vi "SETUPdll.vi"(8 "error in (no error)":errorcluster, 11 "Inputs":T1={"ncomp - Number of Components"=1, "hfld - Fluid/Mixture Components"="", "hfm - Mixture Coefficients "="", "hrf - Reference state"="DEF"}) -> (0 "error out":errorcluster, 2 "herr out":string, 3 "ierr out":i32=101)   [LabVIEW 2021]
doc: "INITIALIZATION SUBROUTINES\n\nsubroutine SETUP (ncomp,hfiles,hfmix,hrf,ierr,herr)\n\ndefine models and initialize arrays\n\nA call to this routine is required.\n\nINPUTS:\nncomp -- number of components (1 for pure fluid) [integer]\n if called with ncomp=-1, the version number*10000 will be returned in ierr\nhfiles -- array of file names specifying fluid/mixture components\n [character*255 variable] for each of the ncomp components;\n e.g., :fluids:r134a.fld (Mac) or fluids\\r134a.fld (DOS) or\n [full_path]/fluids/r134a.fld (UNIX)\nhfmix -- mixture coefficients [character*255]\n file name containing coefficients for mixture model,\n if applicable\n e.g., fluids\\hmx.bnc\nhrf -- reference state for thermodynamic calculations [character*3]\n 'DEF': default reference state as specified in fluid file\n is applied to each pure component\n 'NBP': h,s = 0 at pure component normal boiling point(s)\n 'ASH': h,s = 0 for sat liquid at -40 C (ASHRAE convention)\n 'IIR': h = 200, s = 1.0 for sat liq at 0 C (IIR convention)\n other choices are possible, but these require a separate\n call to SETREF\nOUTPUTS:\nierr -- error flag: 0 = successful\n 101 = error in opening file\n 102 = error in file or premature end of file\n -103 = unknown model encountered in file\n 104 = error in setup of model\n 105 = specified model not found\n 111 = error in opening mixture file\n 112 = mixture file of wrong type\n 114 = nc<>nc from setmod\n -117 = binary pair not found, all parameters will be estimated\n 117 = No mixture data are available, mixture is outside the\n range of the model and calculations will not be made\nherr -- error string (character*255 variable if ierr<>0)\n [fluid parameters, etc. returned via various common blocks]\nhfld_length -- length of variable hfld (default: 10000)\nhfm_length -- length of variable hfm (default: 255)\nhrf_length -- length of variable hrf (default: 3)\nherr_length -- : length of variable herr (default: 255)"
uses:
  REFPROP.dll
panel:
  # "REFPROP-SETUP_dll.vi"
  # "void  SETUPdll(int32_t *ncomp, CStr hfiles, CStr hfmix, CStr hrf, int32_t *ierr, CStr herr, int32_t hfile_Lengh, int32_t hfmix_length, int32_t hrf_length, int32_t herr_length)"
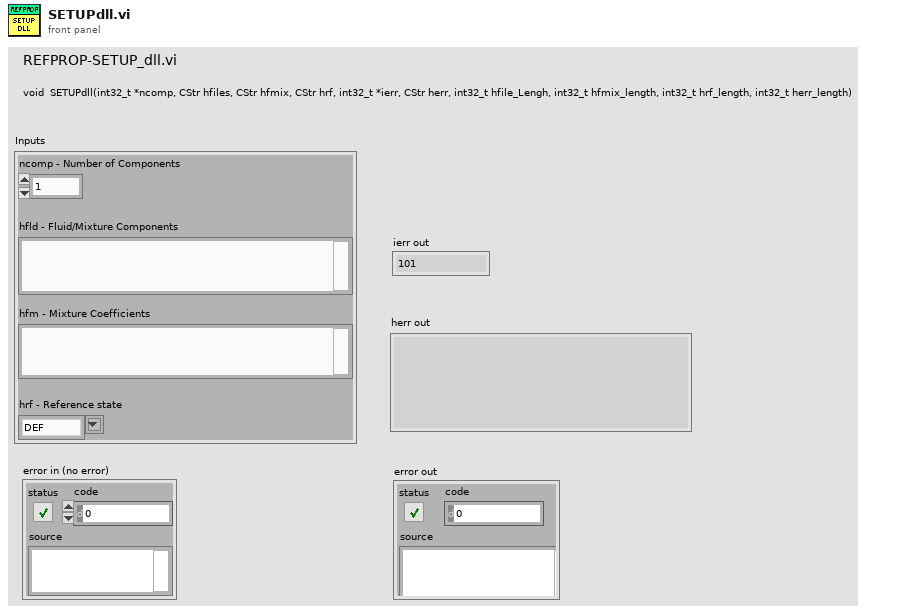
[diagram p1: front panel]
types:
  T1 = cluster{"ncomp - Number of Components":i32, "hfld - Fluid/Mixture Components":string, "hfm - Mixture Coefficients ":string, "hrf - Reference state":string}
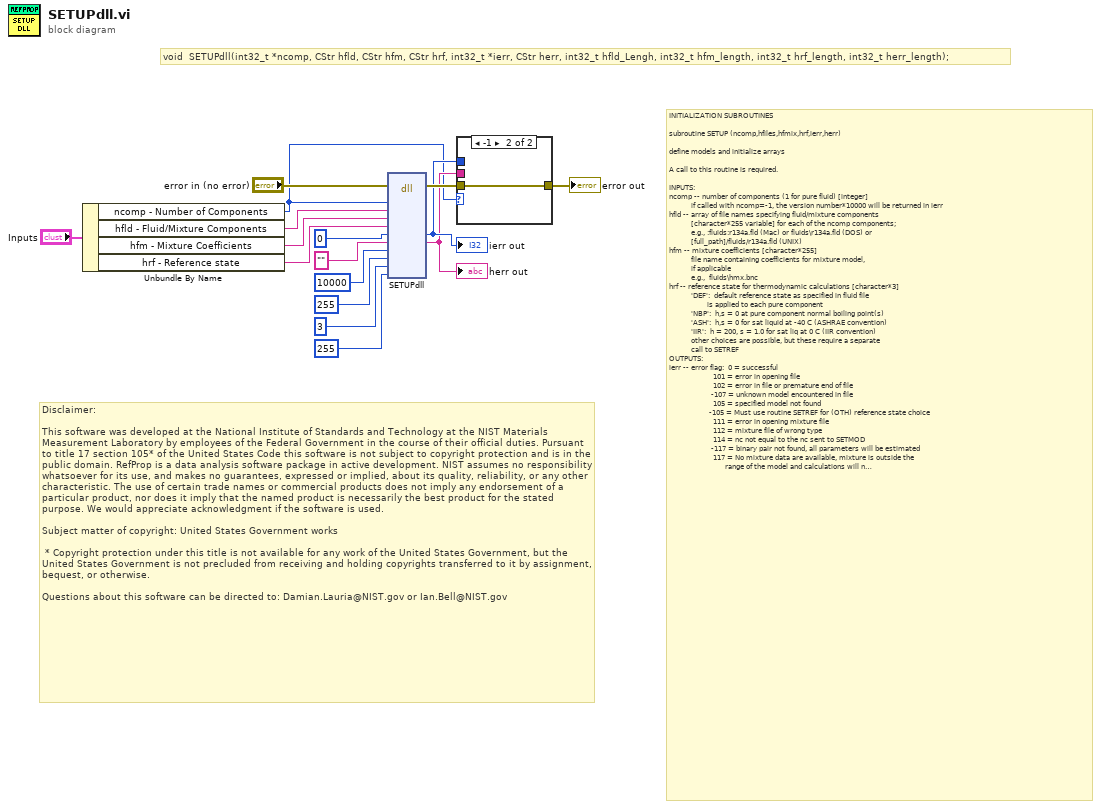
[diagram p0: block diagram]
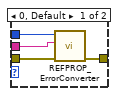
[diagram p2: hidden frame]
diagram:
  # "Disclaimer:\n\nThis software was developed at the National Institute of Standards and Technology at the NIST Materials Measurement Laboratory by employees of the Federal Government in the course of their official duties. Pursuant to title 17 section 105* of the United States Code this software is not subject to copyright protection and is in the public domain. RefProp is a data analysis software package in active development. NIST assumes no responsibility whatsoever for its use, and makes no guarantees, expressed or implied, about its quality, reliability, or any other characteristic. The use of certain trade names or commercial products does not imply any endorsement of a particular product, nor does it imply that the named product is necessarily the best product for the stated purpose. We would appreciate acknowledgment if the software is used.\n \nSubject matter of copyright: United States Government works\n  \n * Copyright protection under this title is not available for any work of the United States Government, but the United States Government is not precluded from receiving and holding copyrights transferred to it by assignment, bequest, or otherwise.\n\nQuestions about this software can be directed to: Damian.Lauria@NIST.gov or Ian.Bell@NIST.gov"
  # "void  SETUPdll(int32_t *ncomp, CStr hfld, CStr hfm, CStr hrf, int32_t *ierr, CStr herr, int32_t hfld_Lengh, int32_t hfm_length, int32_t hrf_length, int32_t herr_length);"
  # "INITIALIZATION SUBROUTINES\n\nsubroutine SETUP (ncomp,hfiles,hfmix,hrf,ierr,herr)\n\ndefine models and initialize arrays\n\nA call to this routine is required.\n\nINPUTS:\nncomp -- number of components (1 for pure fluid) [integer]\n           if called with ncomp=-1, the version number*10000 will be returned in ierr\nhfld -- array of file names specifying fluid/mixture components\n           [character*255 variable] for each of the ncomp components;\n           e.g., :fluids:r134a.fld (Mac) or fluids\\r134a.fld (DOS) or\n           [full_path]/fluids/r134a.fld (UNIX)\nhfm -- mixture coefficients [character*255]\n           file name containing coefficients for mixture model,\n           if applicable\n           e.g.,  fluids\\hmx.bnc\nhrf -- reference state for thermodynamic calculations [character*3]\n           'DEF':  default reference state as specified in fluid file\n                   is applied to each pure component\n           'NBP':  h,s = 0 at pure component normal boiling point(s)\n           'ASH':  h,s = 0 for sat liquid at -40 C (ASHRAE convention)\n           'IIR':  h = 200, s = 1.0 for sat liq at 0 C (IIR convention)\n           other choices are possible, but these require a separate\n           call to SETREF\nOUTPUTS:\nierr -- error flag:  0 = successful\n                      101 = error in opening file\n                      102 = error in file or premature end of file\n                     -107 = unknown model encountered in file\n                      105 = specified model not found\n                    -105 = Must use routine SETREF for (OTH) reference state choice \n                      111 = error in opening mixture file\n                      112 = mixture file of wrong type\n                      114 = nc not equal to the nc sent to SETMOD\n                     -117 = binary pair not found, all parameters will be estimated\n                      117 = No mixture data are available, mixture is outside the\n                            range of the model and calculations will not be made\nherr -- error string (character*255 variable if ierr<>0)\n     [fluid parameters, etc. returned via various common blocks]\nhfld_length -- length of variable hfld (default: 10000)\nhfm_length -- length of variable hfm (default: 255)\nhrf_length --  length of variable hrf (default: 3)\nherr_length -- : length of variable herr (default: 255)"
  n1 = Unbundle By Name("Inputs") -> ("ncomp - Number of Components"=w4:i32, "hfld - Fluid/Mixture Components"=w3:string, "hfm - Mixture Coefficients"=w2:string, "hrf - Reference state"=w1:string)
  n2 = dll-call lib="C:/Users/lauria/OneDrive - National Institute of Standards and Technology (NIST)/LabVIEW Projects/7 REFPROP/REFPROP-wrappers-master/REFPROP-wrappers-master/wrappers/Labview/REFPROP/REFPROP.*" fn="SETUPdll"(error in="error in (no error)", "ncomp"=w4, "hfiles"=w3, "hfmix"=w2, "hrf"=w1, "ierr"=0, "herr"="", "hfiles_Lengh"=10000 ("ln1"), "hfmix_length"=255 ("ln2"), "hrf_length"=3 ("ln3"), "herr_length"=255 ("ln4")) -> (error out=w10:errorcluster, "ierr"=w9:i32, "herr"=w8:string)  [unwired: 11 in, 1 out]
  "ierr out" <- w9
  "herr out" <- w8
  n3 = case shown="-1" w4 {
    tunnel: w10 -> [w20 w21]
    tunnel: [w19 w21] -> w6
    tunnel: w9 -> [w18 _]
    tunnel: w8 -> [w17 _]
    frame 0, Default {
      n4 = call "REFPROP_ErrorConverter.vi"("error in (no error)"=w20, "Error Message"=w17, "Error Code"=w18) -> ("error out"=w19:errorcluster)  [unwired: 8 in]
    }
    frame -1 {
    }
  }
  "error out" <- w6
